vi "_FPGA_Accumulator_30bits.vi"(8 "Reset":bool, 9 "Cycle shift":fxp<+,30,30>, 10 "DeCycle":fxp<+,30,30>, 11 "Enable (Clk)":bool) -> (2 "Output":fxp<+,32,32>)   [LabVIEW 2018]
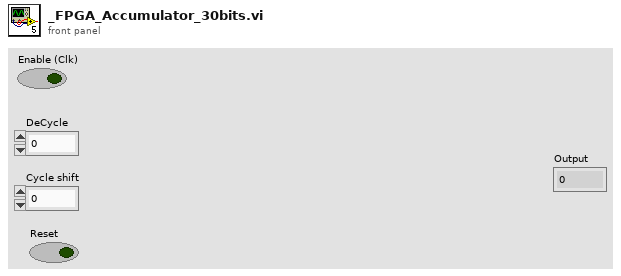
[diagram p1: front panel]
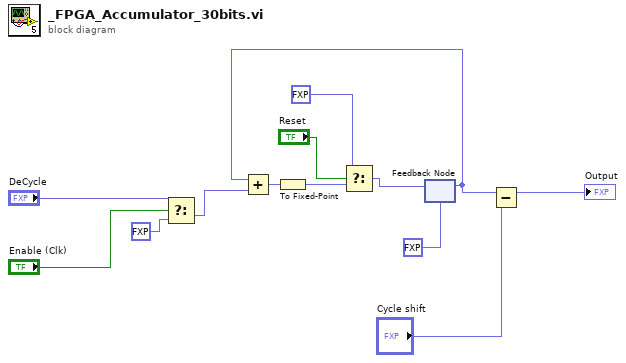
[diagram p0: block diagram]
diagram:
  n1 = Select(t="DeCycle", s="Enable (Clk)", f=fxp<+,30,30> 0.0) -> (s? t:f=w10:fxp<+,30,30>)
  n2 = feedback #1(fxp<+,30,30> 0.0) -> (w12:fxp<+,30,30>)
  n3 = Add(x=w12, y=w10) -> (x+y=w13:fxp<+,32,32>)
  n4 = To Fixed-Point(number=w13) -> (fixed-point=w5:fxp<+,30,30>)  [unwired: 1 in]
  n5 = Select(t=fxp<+,30,30> 0.0, s="Reset", f=w5) -> (s? t:f=w6:fxp<+,30,30>)
  n6 = feedback-in #1(w6) -> ()
  n7 = Subtract(x=w12, y="Cycle shift") -> (x-y=→"Output":fxp<+,32,32>)
